vi "test_TxUDP-RxUDP - Multiple Boards - Many Channels.vi"(8 "error in":errorcluster, 11 "reference in":refnum<class "AIM ARINC 664 Loopback.lvclass">) -> (0 "error out":errorcluster, 3 "reference out":refnum<class "AIM ARINC 664 Loopback.lvclass">)   [LabVIEW 2020, in "AIM ARINC 664 Loopback.lvclass"]
uses:
  AIM ARINC 664 Loopback.lvclass
  C:/Program Files (x86)/National Instruments/LabVIEW 2020/vi.lib/NI/VeriStand Custom Device Testing Tools/VeriStandTestCase/VeriStandTestCase.lvclass
  AIM ARINC 664 Loopback.lvclass/AIM ARINC 664 Loopback.ctl
  NationalInstruments.VeriStand.SystemDefinitionAPI
  b47c41b5-a02e-49d5-b852-4e28f097d7ad.vi
  6a3dd3ed-914d-4d14-bf18-724521aa5e28.vi
  8abe1e9f-12f7-4d29-bb0e-ea5e1950c3f4.vi
  <vilib>/addons/_JKI Toolkits/VI Tester/TestCase.llb/TestCase.lvclass
  Scripting/AIM ARINC 664 Scripting.lvlib
  Import/AIM ARINC 664 Import.lvlib
  <vilib>/NI/VeriStand Custom Device Testing Tools/VeriStandTestCase/VeriStandTestCase.lvclass
  C:/Program Files (x86)/National Instruments/LabVIEW 2020/vi.lib/addons/_JKI Toolkits/VI Tester/TestCase.llb/TestCase.lvclass
panel:
  out "resulting string":string
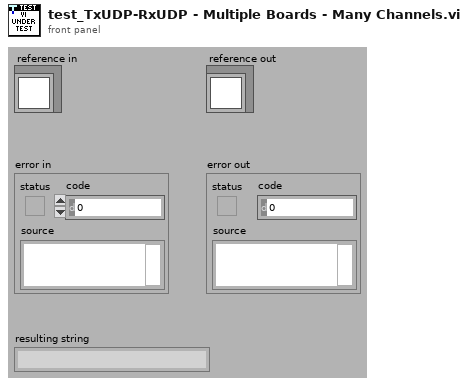
[diagram p1: front panel]
types:
  T1 = typedef "Custom Device API.lvlib/Custom Device Item Ref.ctl" = u64
  T2 = typedef "AIM ARINC 664 Import.lvlib/Board Top Level Configuration.ctl" = cluster{"boardSetup":T3, "portConfiguration":T4[]}
  T3 = typedef "AIM ARINC 664 Import.lvlib/board_setup.ctl" = cluster{"boardId":u32, "portSpeed":u32, "portConfig":u32}
  T4 = typedef "AIM ARINC 664 Import.lvlib/port_configuration.ctl" = cluster{"portSetup":T5, "Tx_Generic":T6[], "Rx_Monitor":cluster{"DefaultCronoMode":u32, "GlbMonBufferSizeIn":u32, "CaptureMode":u32, "MaxFileSizeMB":u32, "Strobe":u32, "TriggerPosition":u32}[], "Tx_UDP":cluster{"tx_udp_setup":cluster{"VlId":i32, "Bag":i32, "NetSelect":u32, "domainID":u8, "sideID":u8, "locationID":u8, "interfaceID":u8, "NumOfSubVl":u16, "Skew":u32, "MaxFrameLength":u32, "FrameBufferSize":u32}, "commPorts":T10[], "sapPorts":T14[]}[], "Rx_UDP":cluster{"Tx_UDP":T15, "commPorts":T16[], "sapPorts":T17[]}[]}
  T5 = typedef "AIM ARINC 664 Import.lvlib/port_setup.ctl" = cluster{"port Id":u32, "redundant":bool}
  T6 = typedef "AIM ARINC 664 Import.lvlib/session_tx_generic.ctl" = cluster{"tx_generic_setup":T7, "Frame Headers":cluster{"ID":string, "Frame header":cluster{"FrameStartMode":i32, "InterFrameGap":i32, "PacketGroupWaitTime":i32, "NetSelect":u32, "PayloadBufferMode":i32, "PayloadGenerationMode":i32, "PhysErrorInjection":i32, "PreambleCount":i32, "SequenceNumberInit":T8, "SequenceNumberOffset":T9, "Skew":i32}}[]}
  T7 = typedef "AIM ARINC 664 Import.lvlib/tx_generic_setup.ctl" = cluster{"QueueSizeIn":u32, "Count":i32, "StartMode":i32}
  T8 = typedef "AIM ARINC 664 Import.lvlib/frame_tx_generic_seqNumberInit.ctl" = i32
  T9 = typedef "AIM ARINC 664 Import.lvlib/frame_tx_generic_seqNumberOffset.ctl" = i32
  T10 = typedef "AIM ARINC 664 Import.lvlib/port_tx_udp_comm.ctl" = cluster{"ID":string, "partitionID":u8, "UdpSrcPort":u16, "UdpDstPort":u16, "PortType":enum16{"FDX_UDP_SAMPLING", "FDX_UDP_QUEUING"}, "SubVIId":u32, "UdpNumBufMessages":u32, "UdpMaxMessageSize":u32, "UdpSamplingRate":u32, "Parameters":T11[]}
  T11 = typedef "AIM ARINC 664 Import.lvlib/frame_parameter.ctl" = cluster{"name":string, "default value":dbl, "unit":string, "Parameter":T12}
  T12 = typedef "AIM ARINC 664 Import.lvlib/frame_parameter_definition.ctl" = cluster{"start index":i32, "size":i32, "encoding":T13, "signed":bool, "scale multiplier":dbl, "scale offset":dbl}
  T13 = typedef "Encoding and Decoding.lvlib/Encoding.ctl" = enum16{"BNR", "BCD", "Discrete"}
  T14 = typedef "AIM ARINC 664 Import.lvlib/port_tx_udp_sap.ctl" = cluster{"ID":string, "SubVlId":u8, "UdpSrcPort":u16, "UdpNumBufMessages":u32, "UdpMaxMessageSize":u32, "partitionID":u8, "domainID":u8, "sideID":u8, "locationID":u8, "interfaceID":u8, "Parameters":T11[]}
  T15 = typedef "AIM ARINC 664 Import.lvlib/rx_udp_setup.ctl" = cluster{"VerificationMode":u32, "Bag":u32, "Jitter":u32, "MaxFrameLength":u32, "MaxSkew":u32, "VLBufSize":u32, "FilterMode":u32, "FilterPosition":u32, "Padding":u32, "FilterMask":u32, "FilterData":u32, "MinFrameLength":u32, "VlId":u16, "VLRange":u32}
  T16 = typedef "AIM ARINC 664 Import.lvlib/port_rx_udp_comm.ctl" = cluster{"ID":string, "domainID":u8, "sideID":u8, "locationID":u8, "partitionID":u8, "UdpSrcPort":u16, "UdpDstPort":u16, "PortType":enum16{"FDX_UDP_SAMPLING", "FDX_UDP_QUEUING"}, "SubVIId":u32, "UdpNumBufMessages":u32, "UdpMaxMessageSize":u32, "UdpSamplingRate":u32, "Parameters":T11[]}
  T17 = typedef "AIM ARINC 664 Import.lvlib/port_rx_udp_sap.ctl" = cluster{"ID":string, "UdpDstPort":u16, "UdpNumBufMessages":u32, "UdpMaxMessageSize":u32, "Parameters":T11[]}
  T18 = typedef "Payload Map.ctl" = map{string, T19}
  T19 = typedef "Payload Record Type.ctl" = cluster{"Data":u8[], "Type of Frame":T20}
  T20 = typedef "Type of Payload.ctl" = u16
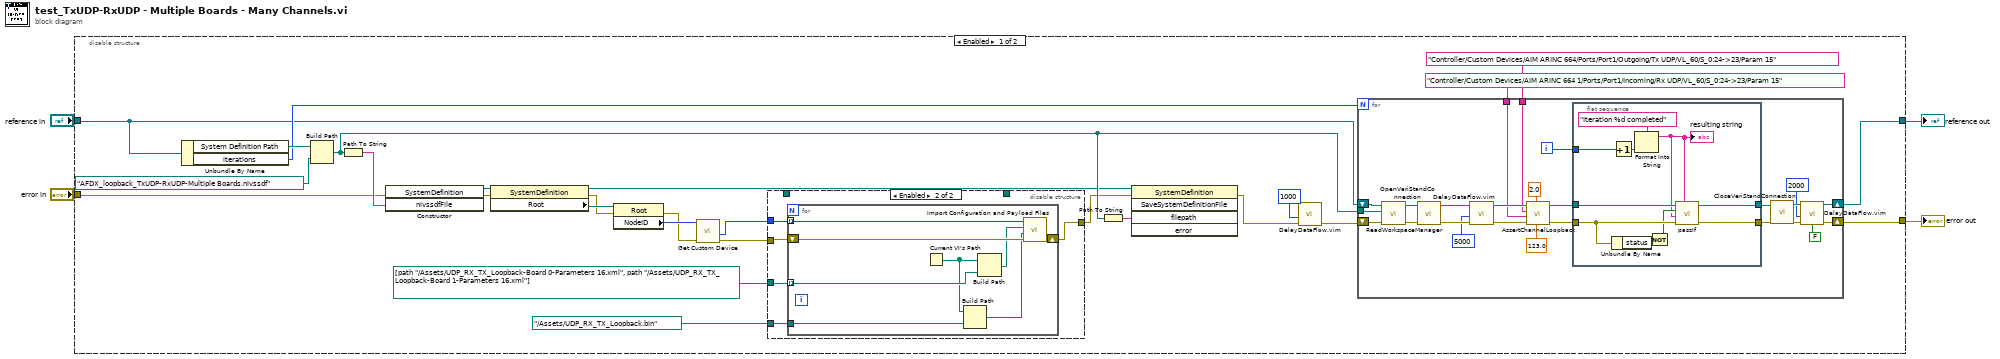
[diagram p0: block diagram]
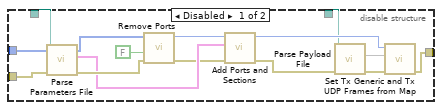
[diagram p2: hidden frame]
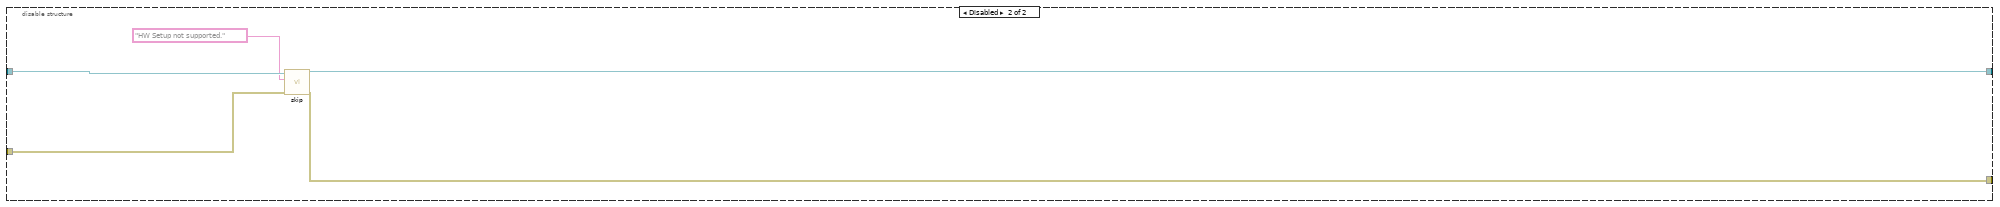
[diagram p3: hidden frame]
diagram:
  n1 = disable-structure shown="Enabled" {
    disable-tunnel: "reference in" -> [w9 w96]
    disable-tunnel: "error in" -> [w8 w95]
    disable-tunnel: [w29 w94] -> w2
    disable-tunnel: [w28 w93] -> w1
    frame Enabled {
      n2 = Unbundle By Name(w9) -> ("System Definition Path"=w31:path, "iterations"=w15:i32)
      n3 = Build Path(base path=w31, name or relative path=path "AFDX_loopback_TxUDP-RxUDP-Multiple Boards.nivssdf") -> (appended path=w26:path)
      n4 = Path To String(path=w26) -> (string=w27:string)
      n5 = constructor class="SystemDefinition"(error in=w8, "nivssdfFile"=w27) -> (reference out=w25:refnum<k24>, error out=w23:errorcluster)  [unwired: 2 in, 2 out]
      n6 = property class="SystemDefinition"(reference=w25, error in=w23) -> (reference out=w20:refnum<k24>, error out=w22:errorcluster, "Root"=w24:refnum<k24>)
      n7 = property class="Root"(reference=w24, error in=w22) -> (error out=w17:errorcluster, "NodeID"=w18:u64)  [unwired: 1 out]
      n8 = call "Get Custom Device.vi"("error in"=w17, "custom device ref in"=w18) -> ("error out"=w16:errorcluster, "Item Refs"=w7:T1[])  [unwired: 5 in, 3 out]
      n9 = disable-structure shown="Enabled" {
        disable-tunnel: w7 -> [w77 w82]
        disable-tunnel: w16 -> [w69 w83]
        disable-tunnel: _ -> [w67 _]
        disable-tunnel: _ -> [w66 _]
        disable-tunnel: [w65 w81] -> w21
        disable-tunnel: path[] [path "../Assets/UDP_RX_TX_Loopback-Board 0-Parameters 16.xml", path "../Assets/UDP_RX_TX_Loopback-Board 1-Parameters 16.xml"] -> [_ w80]
        disable-tunnel: path "../Assets/UDP_RX_TX_Loopback.bin" -> [_ w79]
        frame Disabled {
          n10 = call "Parse Parameters File.vi"("error in"=w69, "path to XML document"=w66) -> ("error out"=w78:errorcluster, "board configuration out"=w75:T2)  [unwired: 7 in, 1 out]
          n11 = call "Remove Ports.vi"("error in"=w78, "refresh?"=FALSE, "Custom device Ref"=w77) -> ("error out"=w74:errorcluster, "Custom device Ref out"=w76:T1)  [unwired: 7 in]
          n12 = call "Add Ports and Sections.vi"("error in"=w74, "board configuration in"=w75, "custom device ref"=w76) -> ("error out"=w73:errorcluster, "custom device ref out"=w68:T1)  [unwired: 7 in]
          n13 = call "Parse Payload File.vi"("error in"=w73, "frame array path in"=w67) -> ("error out"=w72:errorcluster, "Map"=w71:T18)  [unwired: 7 in, 1 out]
          n14 = call "Set Tx Generic and Tx UDP Frames from Map.vi"("error in"=w72, "payload map"=w71, "custom device ref"=w68) -> ("error out"=w65:errorcluster)  [unwired: 7 in, 1 out]
        }
        frame Enabled {
          n15 = for {
            shift-right: [w90] -> w81
            shift-left: w83 -> [w91]
            tunnel: w80 -> [w87] mode=indexing
            tunnel: w82 -> [w86] mode=indexing
            tunnel: w79 -> [w84]
            n16 = Current VI's Path() -> (path=w85:path)
            n17 = Build Path(base path=w85, name or relative path=w84) -> (appended path=w89:path)
            n18 = Build Path(base path=w85, name or relative path=w87) -> (appended path=w88:path)
            n19 = call "Import Configuration and Payload Files.vi"("error in"=w91, "payload file path"=w89, "parameters configuration file path"=w88, "custom device ref"=w86) -> ("error out"=w90:errorcluster)  [unwired: 6 in, 1 out]
          }
        }
      }
      n20 = Path To String(path=w26) -> (string=w19:string)
      n21 = invoke class="SystemDefinition" method="SaveSystemDefinitionFile"(reference=w20, error in=w21, "filepath"=w19) -> (error out=w14:errorcluster)  [unwired: 2 in, 4 out]
      n22 = call "DelayDataFlow.vim"("value in"=w14, "milliseconds to wait"=u32 1000) -> ("value out"=w13:errorcluster)  [unwired: 2 in, 1 out]
      n23 = for {
        N: w15 -> [_]
        tunnel: w26 -> [w47]
        shift-right: [w52] -> w28
        shift-left: w9 -> [w54]
        shift-right: [w41] -> w29
        shift-left: w13 -> [w48]
        tunnel: "Controller/Custom Devices/AIM ARINC 664 1/Ports/Port1/Incoming/Rx UDP/VL_60/S_0:24->23/Param 15" -> [w33]
        tunnel: "Controller/Custom Devices/AIM ARINC 664/Ports/Port1/Outgoing/Tx UDP/VL_60/S_0:24->23/Param 15" -> [w32]
        i -> [w35]
        n24 = call-dynamic "OpenVeriStandConnection.vi"("error in (no error)"=w48, "System Definition File"=w47, "VeriStand Test Case in"=w54) -> ("error out"=w53:errorcluster, "VeriStand Test Case out"=w51:refnum<class "AIM ARINC 664 Loopback.lvclass">)  [unwired: 6 in, 1 out]
        n25 = call-dynamic "ReadWorkspaceManager.vi"("error in (no error)"=w53, "VeriStand Test Case in"=w51) -> ("error out"=w50:errorcluster, "VeriStand Test Case out"=w45:refnum<class "AIM ARINC 664 Loopback.lvclass">)  [unwired: 7 in, 1 out]
        n26 = call "DelayDataFlow.vim"("value in"=w50, "milliseconds to wait"=u32 5000) -> ("value out"=w46:errorcluster)  [unwired: 2 in, 1 out]
        n27 = call <vilib>:"AssertChannelLoopback.vi"("Value"=123.0, "Timeout (1 second)"=2.0, "error in (no error)"=w46, "Read Channel"=w33, "Write Channel"=w32, "VeriStand Test Case in"=w45) -> ("error out"=w36:errorcluster, "VeriStand Test Case out"=w34:refnum<class "AIM ARINC 664 Loopback.lvclass">)  [unwired: 4 in]
        n28 = flat-sequence {
          tunnel: [w64] -> w38
          tunnel: [w63] -> w37
          tunnel: w36 -> [w62]
          tunnel: w35 -> [w58]
          tunnel: w34 -> [w56]
          frame #0 {
            n29 = Unbundle By Name(w62) -> ("status"=w61:bool)
            n30 = Increment(x=w58) -> (x+1=w57:i32)
            n31 = Format Into String(format string="Iteration %d completed", w57) -> (resulting string=w55:string)  [unwired: 2 in, 1 out]
            "resulting string" <- w55
            n32 = Not(x=w61) -> (.not. x?=w60:bool)
            n33 = call-dynamic "passIf.vi"("custom report message (\"\")"=w55, "error in (no error)"=w62, "message (\"\")"=w55, "pass"=w60, "TestCase in"=w56) -> ("error out"=w63:errorcluster, "TestCase out"=w64:refnum<class "AIM ARINC 664 Loopback.lvclass">)  [unwired: 5 in]
          }
        }
        n34 = call-dynamic "CloseVeriStandConnection.vi"("error in (no error)"=w37, "VeriStand Test Case in"=w38) -> ("error out"=w42:errorcluster, "VeriStand Test Case out"=w52:refnum<class "AIM ARINC 664 Loopback.lvclass">)  [unwired: 8 in]
        n35 = call "DelayDataFlow.vim"("value in"=w42, "milliseconds to wait"=u32 2000, "no delay on error (T)"=FALSE) -> ("value out"=w41:errorcluster)  [unwired: 1 in, 1 out]
      }
    }
    frame Disabled {
      n36 = call <vilib>:"skip.vi"("error in (no error)"=w95, "skipMessage"="HW Setup not supported.", "TestCase in"=w96) -> ("error out"=w94:errorcluster, "TestCase out"=w93:refnum<class "AIM ARINC 664 Loopback.lvclass">)  [unwired: 7 in]
    }
  }
  "error out" <- w2
  "reference out" <- w1
